vi "rvc Generate polynomial for trajectory.vi"(6 "final velocity":dbl, 7 "initial velocity":dbl, 9 "number of points":dbl=50.0, 10 "final position":dbl=1.0, 11 "initial position":dbl) -> (1 "ddcoeff":dbl[](array[numeric]), 2 "dcoeff":dbl[](array[numeric]), 3 "coeff":dbl[](array[numeric]))   [LabVIEW 2017]
uses:
  <vilib>/Analysis/7linalg.llb/Solve Linear Equations (single right hand).vi
  <vilib>/Analysis/baseanly.llb/Solve Linear Equations By Cholesky.vi
  <vilib>/Analysis/baseanly.llb/Real Matrix to Compact Array.vi
  <vilib>/Analysis/baseanly.llb/Real Compact Tri-Matrix Linear Eqs.vi
  <vilib>/Analysis/7linalg.llb/Solve Linear Eqs (General).vi
  <vilib>/Analysis/7linalg.llb/Solve Linear Eqs (Gen, single right hand).vi
  <vilib>/Analysis/polynomials.llb/nth Derivative of Polynomial (DBL).vi
  <vilib>/addons/Control Design/_Model Construction/NI_LinSys_Model Creation.lvlib
  <vilib>/Analysis/NI_AALPro.lvlib
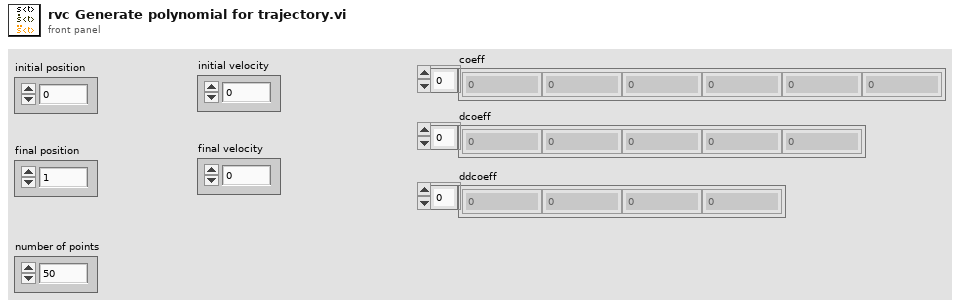
[diagram p1: front panel]
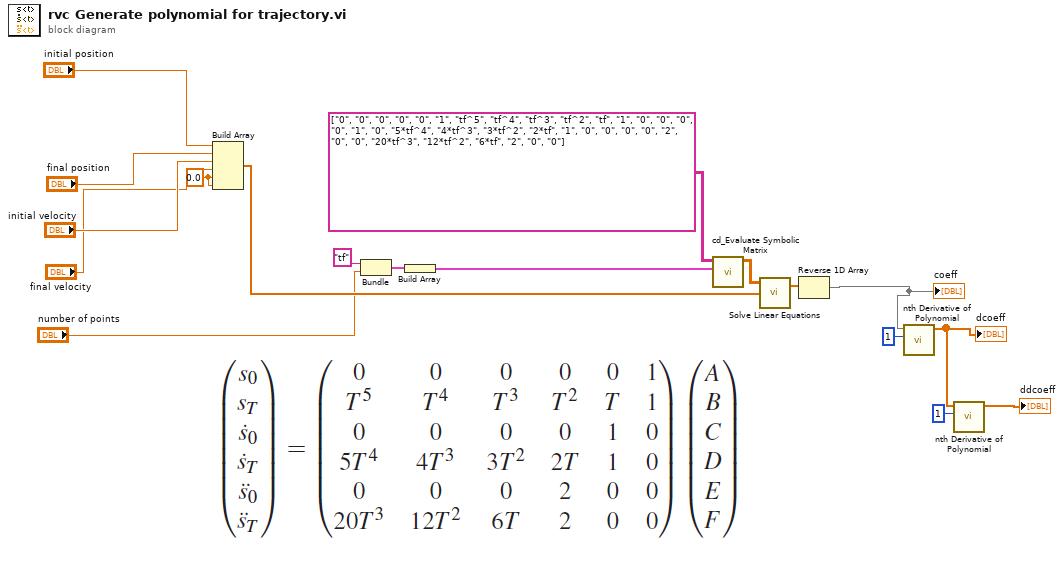
[diagram p0: block diagram]
diagram:
  w11 = 0.0 ("element")
  n1 = Build Array("initial position", "final position", "initial velocity", "final velocity", w11, w11) -> (w10:dbl[])
  n2 = Bundle("Name"="tf", "number of points"="number of points") -> (w17:cluster{"Name":string, "number of points":dbl})  [unwired: 1 in]
  n3 = Build Array(w17) -> (w16:cluster{"Name":string, "number of points":dbl}[])
  n4 = call <vilib>:"cd_Evaluate Symbolic Matrix.vi"("Variables"=w16, "Symbolic Matrix"=string[][] [["0", "0", "0", "0", "0", "1"], ["tf^5", "tf^4", "tf^3", "tf^2", "tf", "1"], ["0", "0", "0", "0", "1", "0"], ["5*tf^4", "4*tf^3", "3*tf^2", "2*tf", "1", "0"], ["0", "0", "0", "2", "0", "0"], ["20*tf^3", "12*tf^2", "6*tf", "2", "0", "0"]]) -> ("Numeric Matrix"=w2:dbl[][])  [unwired: 8 in, 1 out]
  n5 = call-poly <vilib>:"Solve Linear Equations.vi"("Known Vector"=w10, "Input Matrix"=w2) -> ("Solution Vector"=w3:dbl[])  [unwired: 1 in, 1 out]
  n6 = Reverse 1D Array(array=w3) -> (reversed array=w1:dbl[])
  "coeff" <- w1
  n7 = call-poly <vilib>:"nth Derivative of Polynomial.vi"("order"=1, "P(x)"=w1) -> ("Nth Derivative of P(x)"=w6:dbl[])  [unwired: 8 in, 1 out]
  "dcoeff" <- w6
  n8 = call-poly <vilib>:"nth Derivative of Polynomial.vi"("order"=1, "P(x)"=w6) -> ("Nth Derivative of P(x)"=→"ddcoeff":dbl[])  [unwired: 8 in, 1 out]
